vi "drawString.vi"(7 "font file":path, 8 "input buffer":u8[](array[numeric]), 9 "input string":string, 10 "y":u8, 11 "x":u8) -> (3 "output buffer":u8[](array[numeric]))   [LabVIEW 2017]
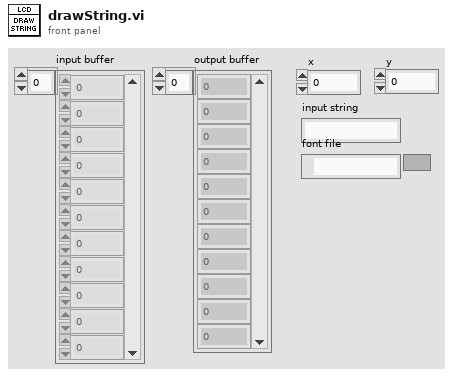
[diagram p1: front panel]
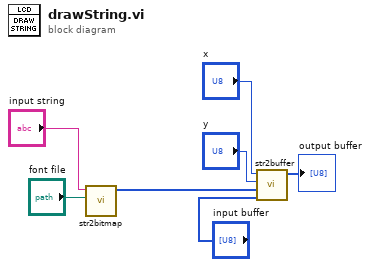
[diagram p0: block diagram]
diagram:
  n1 = call "str2bitmap.vi"("file"="font file", "String"="input string") -> ("bitmap"=w7:u8[])  [unwired: 8 in, 1 out]
  n2 = call "str2buffer.vi"("input buffer"="input buffer", "string bitmap"=w7, "y"="y", "x"="x") -> ("output buffer"=→"output buffer":u8[])  [unwired: 5 in]
